vi "RefreshLoad.vi"(0 "MessageBox":refnum<vi>, 6 "Downsample":i32, 7 "Cluster":T2, 8 "DataPileIn":T1(array[cluster]), 9 "FileList":string[](array[string]), 10 "DEMP Folder":path, 11 "FileListIn":string[](array[string])) -> (1 "dt":dbl, 2 "Channels":string[](array[string]), 3 "DataPile":T1(array[cluster]), 4 "FileList":string[](array[string]), 5 "Keys":string[](array[string]))   [LabVIEW 2024]
uses:
  E:/CodeProjects/DEMPViewer/ClassLibrary1.dll
  ClassLibrary1.dll
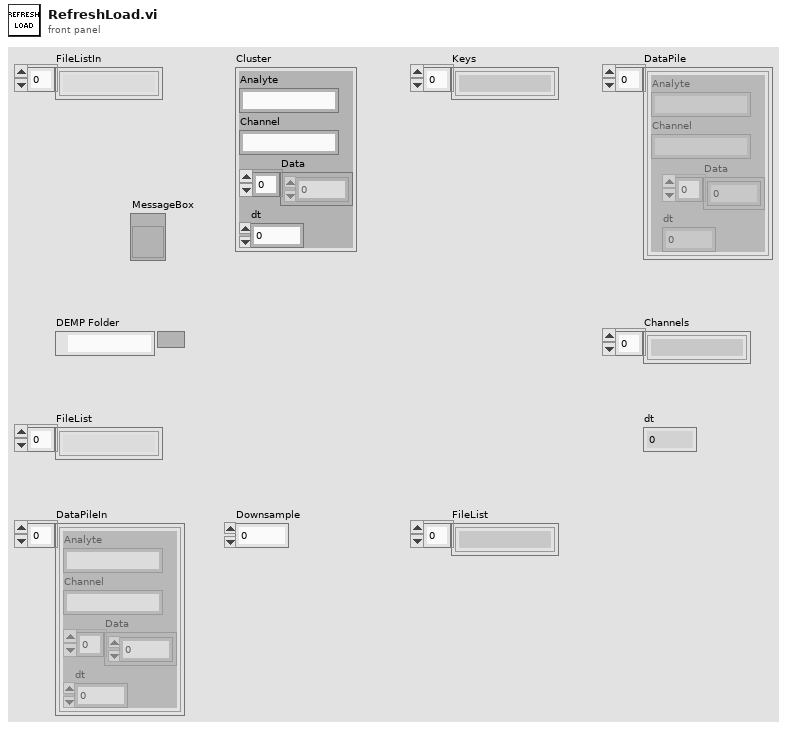
[diagram p1: front panel]
types:
  T1 = cluster{"Analyte":string, "Channel":string, "Data":dbl[], "dt":dbl}[]
  T2 = cluster{"Analyte":string, "Channel":string, "Data":dbl[], "dt":dbl}
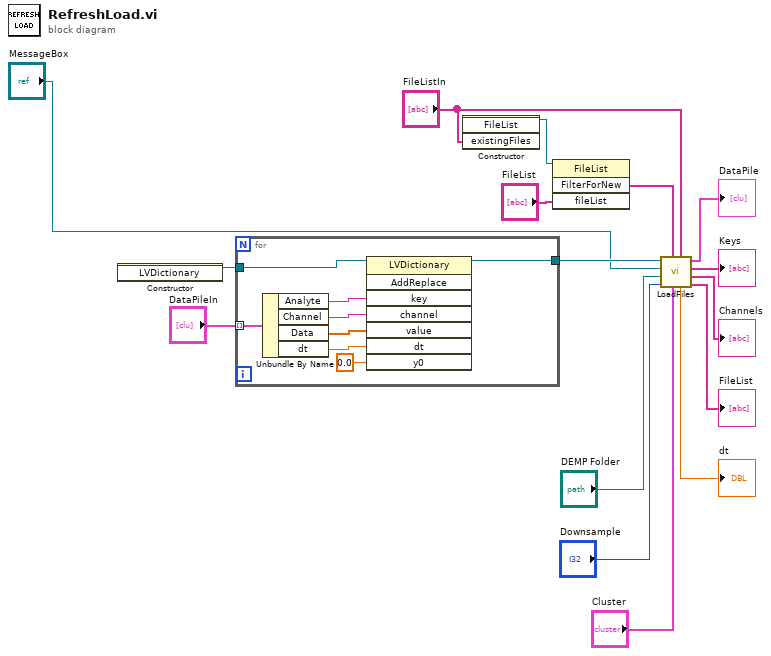
[diagram p0: block diagram]
diagram:
  n1 = constructor class="LVDictionary"() -> (reference out=w8:refnum<k24>)  [unwired: 3 in, 2 out]
  n2 = for {
    tunnel: "DataPileIn" -> [w24] mode=indexing
    tunnel: w8 -> [w23]
    tunnel: [w17] -> w7
    n3 = Unbundle By Name(w24) -> ("Analyte"=w22:string, "Channel"=w21:string, "Data"=w20:dbl[], "dt"=w19:dbl)
    n4 = invoke class="LVDictionary" method="AddReplace"(reference=w23, "key"=w22, "channel"=w21, "value"=w20, "dt"=w19, "y0"=0.0) -> (reference out=w17:refnum<k24>)  [unwired: 2 in, 7 out]
  }
  n5 = constructor class="FileList"("existingFiles"="FileListIn") -> (reference out=w5:refnum<k24>)  [unwired: 3 in, 3 out]
  n6 = invoke class="FileList" method="FilterForNew"(reference=w5, "fileList"="FileList") -> ("FilterForNew"=w3:string[])  [unwired: 2 in, 3 out]
  n7 = call "LoadFiles.vi"("FileListIn in"="FileListIn", "Cluster"="Cluster", "FileList"=w3, "Downsample"="Downsample", "DEMP Folder"="DEMP Folder", "MessageBox"="MessageBox", "FileDictionary"=w7) -> ("FileListIn out"=→"FileList":string[], "Channels"=→"Channels":string[], "Keys"=→"Keys":string[], "DataPile"=→"DataPile":T1, "dt"=→"dt":dbl)
